vi "PC_DRVG to DRVM multiple channels no trigger.vi"() -> ()   [LabVIEW 2021]
uses:
  DC-RMS Voltage Measurement/Typedefs/DC and RMS Voltage Measurements.ctl
  DC-RMS Voltage Measurement/Typedefs/Range and Terminal Settings.ctl
  DC-RMS Voltage Measurement/Typedefs/Specific Channel Settings.ctl
  DC Voltage Generation/DAQ_DC Voltage Generation.lvlib
  DC-RMS Voltage Measurement/DAQ_DC-RMS Voltage Measurement.lvlib
panel:
  in  "Range and Terminal Settings":T1={"Global Settings"={"Min Range(V)"=-10.0, "Max Range(V)"=10.0, "Terminal Configuration"=10083}, "Specific Channel Settings"=[{"Active Channels"="Dev1/ai0", "Min Range"=-10.0, "Max Range"=10.0, "Terminal Configuration"=10106}, {"Active Channels"="Dev1/ai1", "Min Range"=-10.0, "Max Range"=10.0, "Terminal Configuration"=10083}]} {"Specific Channel Settings"."Terminal Configuration" items=["RSE"=10083, "NRSE"=10078, "Differential"=10106]; "Specific Channel Settings"."Max Range" format="%.2p"; "Specific Channel Settings"."Min Range" format="%.2p"; "Global Settings"."Terminal Configuration" items=["RSE"=10083, "NRSE"=10078, "Differential"=10106]; "Global Settings"."Max Range(V)" format="%.2p"; "Global Settings"."Min Range(V)" format="%.2p"}
  out "Acquisition Time (s)":dbl=0.1 format="%.2p"
  out "DC Voltage Measurements":T3={"Average DC Voltage (V)"=[4.748138069375946, 3.8193428194796963], "RMS Voltage (V)"=[4.748138079164851, 3.8193428310071993]} {"RMS Voltage (V)" format="%.2p"; "Average DC Voltage (V)" format="%.2p"}
  out "Voltage Waveforms":waveform(dbl)[](graph)=[{"t0"=timestamp(3825153255.788785 s since 1904-01-01), "dt"=9.999999999999999e-05, "Y"=array[1000 elements], "attributes"=variant("NI_ChannelName"=variant(string "Dev1/ai0"), "NI_UnitDescription"=variant(string "Volts"))}, {"t0"=timestamp(3825153255.788796 s since 1904-01-01), "dt"=9.999999999999999e-05, "Y"=array[1000 elements], "attributes"=variant("NI_ChannelName"=variant(string "Dev1/ai1"), "NI_UnitDescription"=variant(string "Volts"))}]
  out "error out":errorcluster
  # "Min. Range(V)"
  # "Max. Range(V)"
  # "Terminal Configuration"
  # "Physical Channel Name"
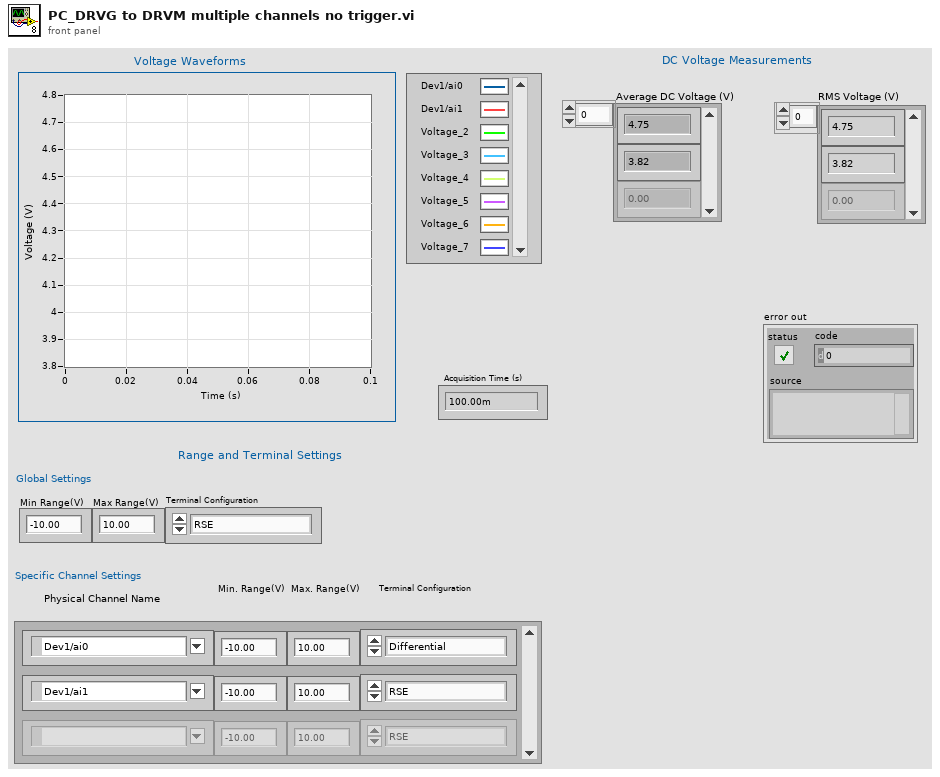
[diagram p1: front panel]
types:
  T1 = typedef "DAQ_DC-RMS Voltage Measurement.lvlib/Range and Terminal Settings.ctl" = cluster{"Global Settings":cluster{"Min Range(V)":dbl, "Max Range(V)":dbl, "Terminal Configuration":i32}, "Specific Channel Settings":T2[]}
  T2 = typedef "DAQ_DC-RMS Voltage Measurement.lvlib/Specific Channel Settings.ctl" = cluster{"Active Channels":tag, "Min Range":dbl, "Max Range":dbl, "Terminal Configuration":i32}
  T3 = typedef "DAQ_DC-RMS Voltage Measurement.lvlib/DC and RMS Voltage Measurements.ctl" = cluster{"Average DC Voltage (V)":dbl[], "RMS Voltage (V)":dbl[]}
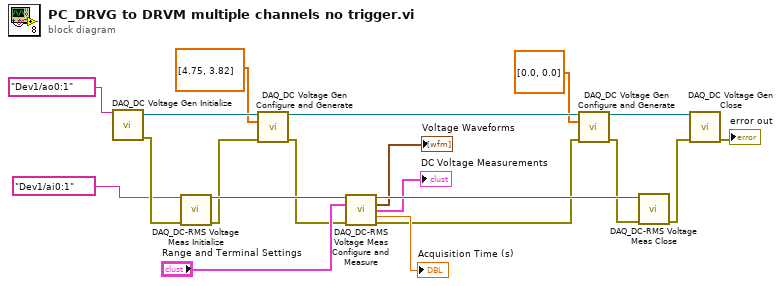
[diagram p0: block diagram]
diagram:
  n1 = call "DAQ_DC Voltage Gen Initialize.vi"("Physical Channels"=tag "Dev1/ao0:1") -> ("DAQmx Task Out"=w20:refnum<k21>, "error out"=w8:errorcluster)  [unwired: 13 in]
  n2 = call "DAQ_DC-RMS Voltage Meas Initialize.vi"("Physical Channels"=tag "Dev1/ai0:1", "error in"=w8) -> ("DAQmx Task Out"=w19:refnum<k21>, "error out"=w7:errorcluster)  [unwired: 12 in]
  n3 = call "DAQ_DC Voltage Gen Configure and Generate.vi"("DAQmx Task In"=w20, "Output Voltages (V)"=dbl[] [4.75, 3.82], "error in"=w7) -> ("DAQmx Task Out"=w17:refnum<k21>, "error out"=w6:errorcluster)  [unwired: 11 in]
  n4 = call "DAQ_DC-RMS Voltage Meas Configure and Measure.vi"("DAQmx Task In"=w19, "Range and Terminal Settings"="Range and Terminal Settings", "error in"=w6) -> ("DAQmx Task Out"=w18:refnum<k21>, "Voltage Waveforms"=→"Voltage Waveforms":waveform(dbl)[], "DC and RMS Voltage Measurements"=→"DC Voltage Measurements":T3, "Acquisition Time (s)"=→"Acquisition Time (s)":dbl, "error out"=w5:errorcluster)  [unwired: 8 in]
  n5 = call "DAQ_DC Voltage Gen Configure and Generate.vi"("DAQmx Task In"=w17, "Output Voltages (V)"=dbl[] [0.0, 0.0], "error in"=w5) -> ("DAQmx Task Out"=w16:refnum<k21>, "error out"=w4:errorcluster)  [unwired: 11 in]
  n6 = call "DAQ_DC-RMS Voltage Meas Close.vi"("DAQmx Task In"=w18, "error in"=w4) -> ("error out"=w3:errorcluster)  [unwired: 13 in]
  n7 = call "DAQ_DC Voltage Gen Close.vi"("DAQmx Task In"=w16, "error in"=w3) -> ("error out"=→"error out":errorcluster)  [unwired: 13 in]
